vi "Auto - Increment State (SubVI).vi"(6 "numberOfBallsShot out":dbl, 8 "disabledRunning":bool, 9 "Auton Cluster In":T1, 11 "Auton State In":i32) -> (1 "Auton cluster Out":T1, 3 "Auton State Out":i32, 4 "End Condition":dbl)   [LabVIEW 2020]
uses:
  TypeDefs/Auton Cluster Typedef.ctl
  Team Code/Robot Global Data.vi
  <vilib>/Rock Robotics/WPI/ThirdParty/JAS_Junk/TrajLib/Trajectory_Library.lvlib
panel:
  # "Inputs"
  # "Outputs"
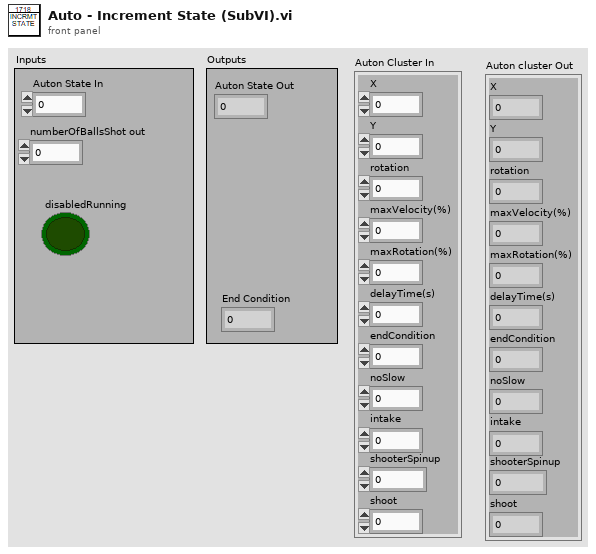
[diagram p1: front panel]
types:
  T1 = typedef "Auton Cluster Typedef.ctl" = cluster{"rotation":dbl, "maxVelocity(%)":dbl, "delayTime(s)":dbl, "endCondition":dbl, "noSlow":dbl, "intake":dbl, "shooterSpinup":dbl, "shoot":dbl, "X":dbl, "Y":dbl, "maxRotation(%)":dbl}
  T2 = typedef "Trajectory_Library.lvlib/SWERVE_DRIVE_ODOMETRY.ctl" = cluster{"POSE":T3, "GyroOffset":T5, "PreviousAngle":T5, "PrevTime":dbl}
  T3 = typedef "Trajectory_Library.lvlib/POSE2D.ctl" = cluster{"TRANSLATION":T4, "ROTATION":T5}
  T4 = typedef "Trajectory_Library.lvlib/TRANSLATION2D.ctl" = cluster{"X":dbl, "Y":dbl}
  T5 = typedef "Trajectory_Library.lvlib/ROTATION2D.ctl" = cluster{"VALUE":dbl, "COS":dbl, "SIN":dbl}
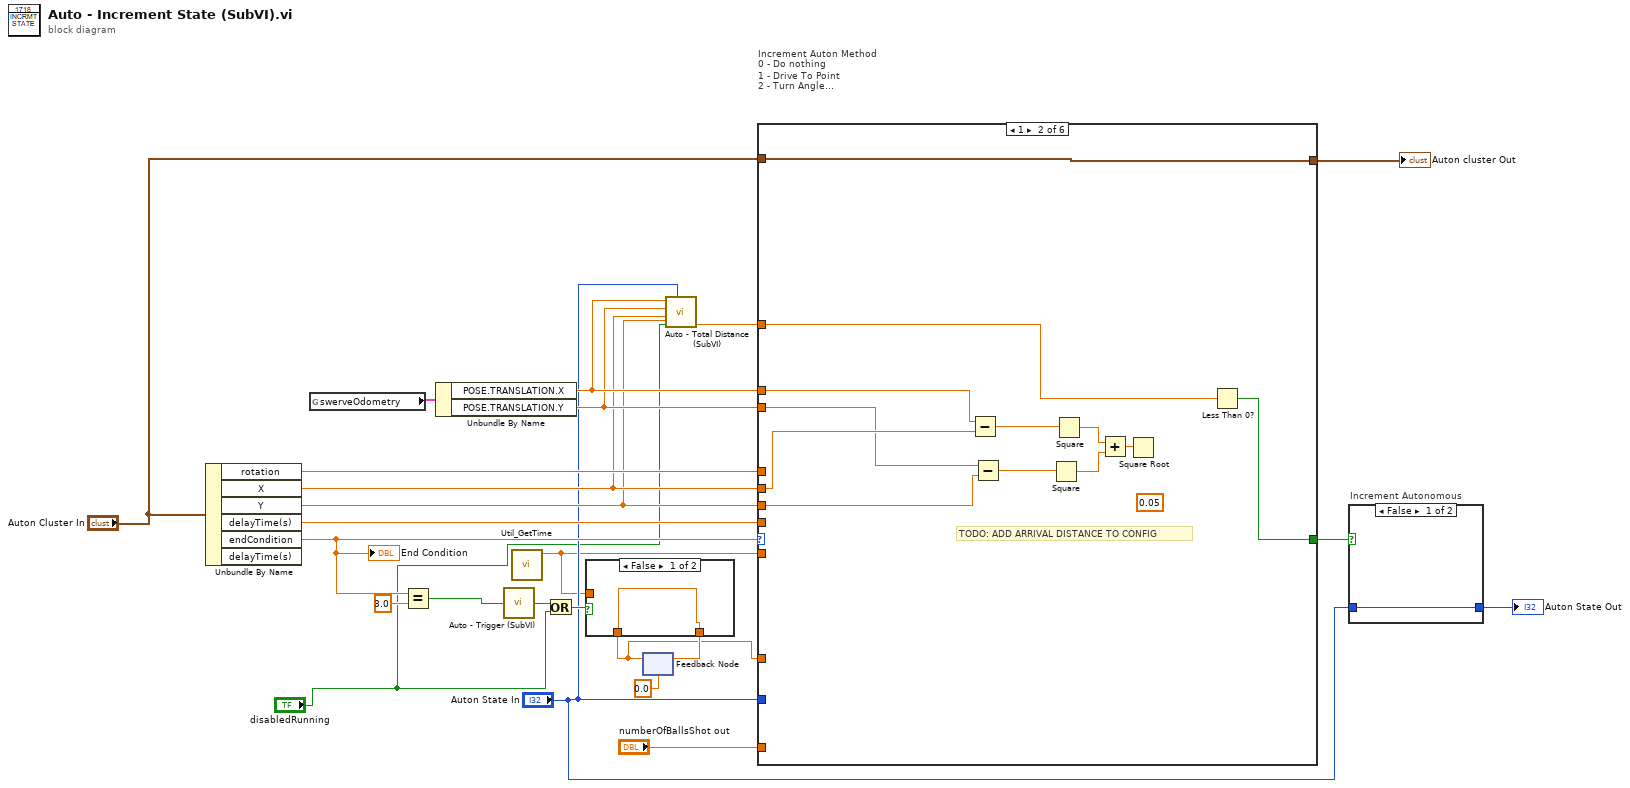
[diagram p0: block diagram]
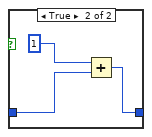
[diagram p3: hidden frame]
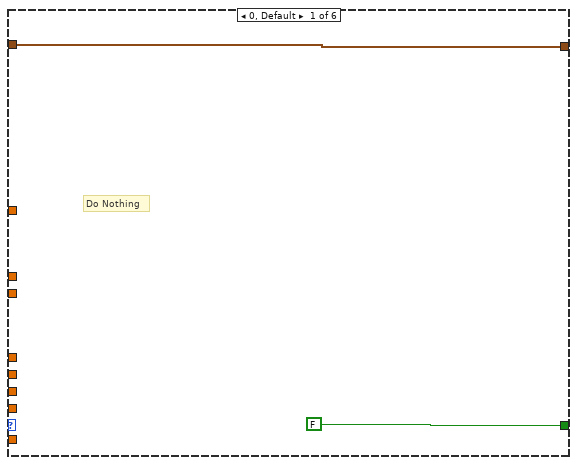
[diagram p4: hidden frame]
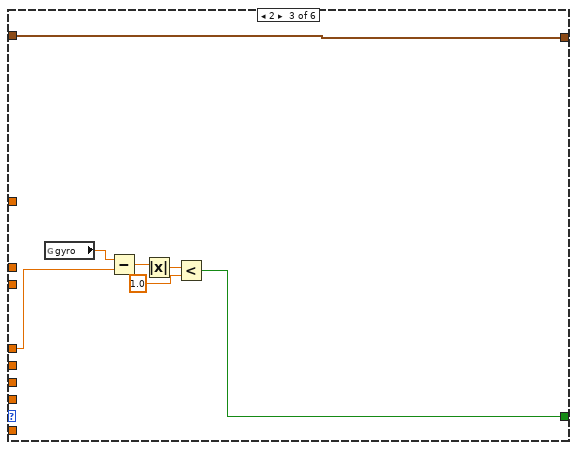
[diagram p5: hidden frame]
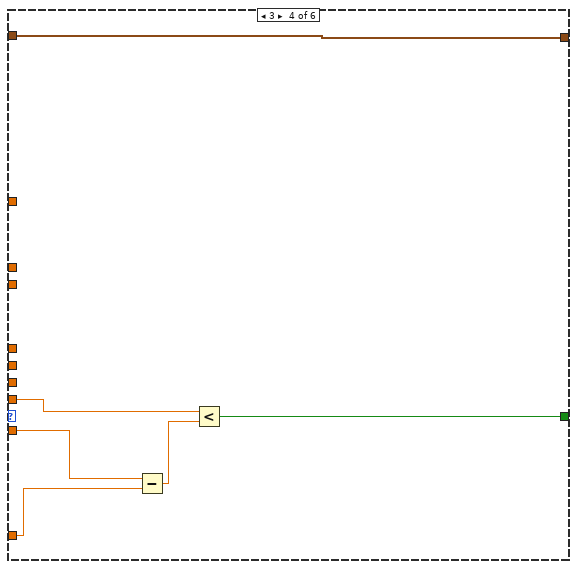
[diagram p6: hidden frame]
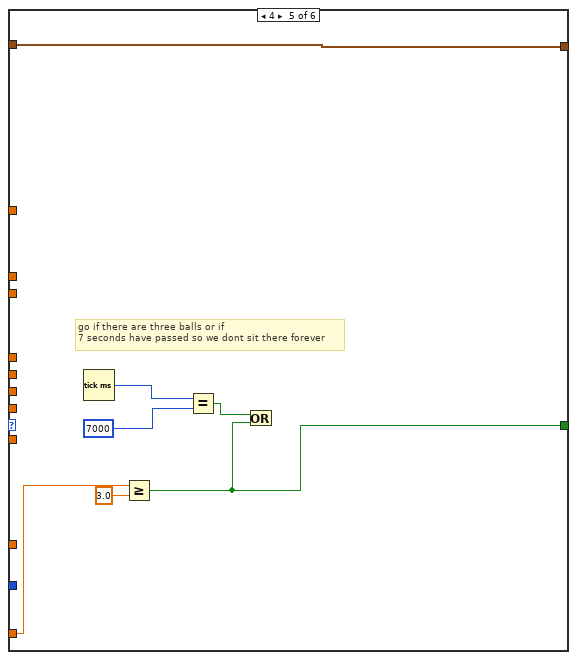
[diagram p7: hidden frame]
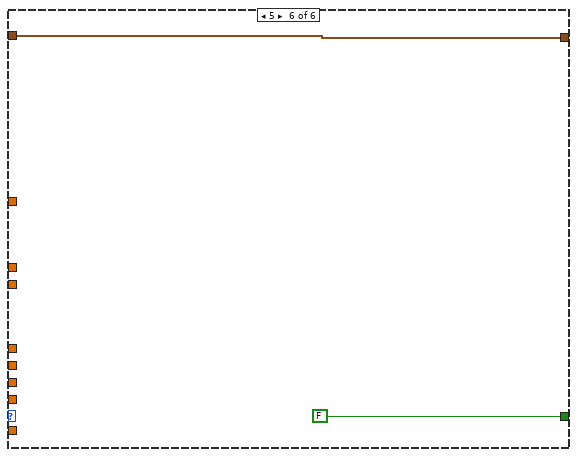
[diagram p8: hidden frame]
diagram:
  n1 = Unbundle By Name("Auton Cluster In") -> ("rotation"=w10:dbl, "X"=w6:dbl, "Y"=w5:dbl, "delayTime(s)"=w22:dbl, "endCondition"=w17:dbl)  [unwired: 1 out]
  "End Condition" <- w17
  n2 = global read "Robot Global Data.vi" "swerveOdometry"() -> (w9:T2)
  n3 = Equal?(x=w17, y=3.0) -> (x = y?=w18:bool)
  n4 = Unbundle By Name(w9) -> ("POSE.TRANSLATION.X"=w8:dbl, "POSE.TRANSLATION.Y"=w7:dbl)
  n5 = call "Auto - Trigger (SubVI).vi"("Trigger"=w18) -> ("Trigger Output"=w13:bool)
  n6 = call <vilib>:"Util_GetTime.vi"() -> ("FPGA_Time_Seconds"=w2:dbl)  [unwired: 10 in, 1 out]
  n7 = Or(x=w13, y="disabledRunning") -> (x .or. y?=w12:bool)
  n8 = feedback #1(0.0) -> (w14:dbl)
  n9 = case shown="False" w12 {
    tunnel: w14 -> [w25 _]
    tunnel: [w25 w26] -> w11
    tunnel: w2 -> [_ w26]
    frame False {
    }
    frame True {
    }
  }
  n10 = feedback-in #1(w11) -> ()
  n11 = call "Auto - Total Distance (SubVI).vi"("Auto Y"=w5, "Auton State In"="Auton State In", "disabledRunning"="disabledRunning", "Auto X"=w6, "Pose Translation Y"=w7, "Pose Translation X"=w8) -> ("distanceLeftToDrivenInThisStep"=w3:dbl)  [unwired: 4 in, 1 out]
  n12 = case "Increment Auton Method\n0 - Do nothing\n1 - Drive To Point\n2 - Turn Angle\n3 - Delay (seconds)\n4 - Number of balls fired (3)\n5 - Turn Turret to Angle" shown="1" w17 {
    tunnel: [FALSE ("Time Expired") w30 w41 w52 w54 FALSE ("Time Expired")] -> w23
    tunnel: w22 -> [_ _ _ w53 _ _]
    tunnel: "Auton Cluster In" -> [w27 w40 w47 w51 w58 w62]
    tunnel: [w27 w40 w47 w51 w58 w62] -> w20
    tunnel: "Auton State In" -> [_ _ _ _ _ _]
    tunnel: "numberOfBallsShot out" -> [_ _ _ _ w60 _]
    tunnel: w6 -> [_ w39 _ _ _ _]
    tunnel: w5 -> [_ w38 _ _ _ _]
    tunnel: w11 -> [_ _ _ w50 _ _]
    tunnel: w10 -> [_ _ w45 _ _ _]
    tunnel: w8 -> [_ w32 _ _ _ _]
    tunnel: w7 -> [_ w31 _ _ _ _]
    tunnel: w3 -> [_ w29 _ _ _ _]
    tunnel: w2 -> [_ _ _ w48 _ _]
    frame 0, Default {
      # "Do Nothing"
    }
    frame 1 {
      (unwired) 0.05 ("y")
      # "TODO: ADD ARRIVAL DISTANCE TO CONFIG"
      n13 = Subtract(x=w32, y=w39) -> (x-y=w34:dbl)
      n14 = Subtract(x=w31, y=w38) -> (x-y=w33:dbl)
      n15 = Square(x=w33) -> (x^2=w36:dbl)
      n16 = Square(x=w34) -> (x^2=w37:dbl)
      n17 = Add(x=w37, y=w36) -> (x+y=w35:dbl)
      n18 = Square Root(x=w35) -> ()  [unwired: 1 out]
      n19 = Less Than 0?(x=w29) -> (x < 0?=w30:bool)
    }
    frame 2 {
      n20 = global read "Robot Global Data.vi" "gyro"() -> (w46:dbl)
      n21 = Subtract(x=w46, y=w45) -> (x-y=w44:dbl)
      n22 = Absolute Value(x=w44) -> (abs(x)=w43:dbl)
      n23 = Less?(x=w43, y=1.0) -> (x < y?=w41:bool)
    }
    frame 3 {
      n24 = Subtract(x=w48, y=w50) -> (x-y=w49:dbl)
      n25 = Less?(x=w53, y=w49) -> (x < y?=w52:bool)
    }
    frame 4 {
      # "go if there are three balls or if \n7 seconds have passed so we dont sit there forever"
      n26 = Tick Count (ms)() -> (millisecond timer value=w57:u32)
      n27 = Greater Or Equal?(x=w60, y=3.0) -> (x >= y?=w54:bool)
      n28 = Equal?(x=w57, y=u32 7000) -> (x = y?=w55:bool)
      n29 = Or(x=w55, y=w54) -> ()  [unwired: 1 out]
    }
    frame 5 {
    }
  }
  "Auton cluster Out" <- w20
  n30 = case "Increment Autonomous" shown="False" w23 {
    tunnel: "Auton State In" -> [w63 w65]
    tunnel: [w63 w66] -> w24
    frame False {
    }
    frame True {
      n31 = Add(x=1, y=w65) -> (x+y=w66:i32)
    }
  }
  "Auton State Out" <- w24
